vi "AlazarBoardsInSystemBySystemID.vi"(0 "System ID":u32, 1 "error in (no error)":errorcluster) -> (2 "Board Count":u32, 3 "Return Code":u32, 4 "error out":errorcluster)   [LabVIEW 2018]
doc: "Return the number of digitizer boards in a board system specified its system ID.s"
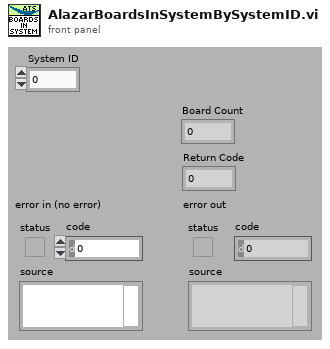
[diagram p1: front panel]
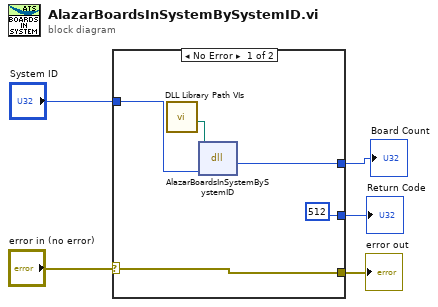
[diagram p0: block diagram]
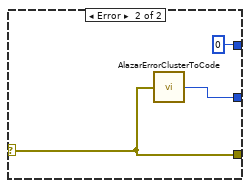
[diagram p2: hidden frame]
diagram:
  n1 = case shown="No Error" "error in (no error)" {
    selector: "error in (no error)" -> [w9 w13]
    tunnel: [w9 w13] -> w4
    tunnel: [u32 512 w12] -> w3
    tunnel: "System ID" -> [w10 _]
    tunnel: [w7 u32 0] -> w1
    frame No Error {
      n2 = call "DLL Library Path VIs.vi"() -> ("Alazar"=w6:path)  [unwired: 9 in, 2 out]
      n3 = dll-call lib="C:/Project/SerialSectOCT - FFT GPU/SerialSectOCT/Labview Software/DLL/ATSApi.dll" fn="AlazarBoardsInSystemBySystemID"(path in=w6, "systemIDs"=w10) -> ("return type"=w7:u32)  [unwired: 3 in, 2 out]
    }
    frame Error {
      n4 = call "AlazarErrorClusterToCode.vi"("error in (no error)"=w13) -> ("Error Code"=w12:u32)
    }
  }
  "error out" <- w4
  "Return Code" <- w3
  "Board Count" <- w1
